vi "Master_continuous.vi"() -> ()   [LabVIEW 2021]
uses:
  Settings.ctl
  Control 2.ctl
  <vilib>/DAQmx/write.llb/DAQmx Write (Digital 1D U32 1Chan NSamp).vi
  <vilib>/DAQmx/create/channels.llb/DAQmx Create Channel (DO-Digital Output).vi
  <vilib>/DAQmx/configure/timing.llb/DAQmx Timing (Sample Clock).vi
  <vilib>/DAQmx/miscellaneous.llb/DAQmx Fill In Error Info.vi
panel:
  in  "stop":bool
  in  "Delay end (ms)":dbl=102.0
  out "# Samples":T1=7800.0 format="%#_9f"
  in  "Sampling Rate (Hz)":T1=100000.0 format="%#_9f"
  out "Blue LED":cluster{i32, dbl, dbl[]}(graph)={0, 1e-05, array[18000 elements]}
  out "EMCCD":cluster{i32, dbl, dbl[]}(graph)={0, 1e-05, array[18000 elements]}
  out "Whisker Cam":cluster{i32, dbl, dbl[]}(graph)={0, 1e-05, array[18000 elements]}
  out "Red LED":cluster{i32, dbl, dbl[]}(graph)={0, 1e-05, array[18000 elements]}
  out "Amber LED":cluster{i32, dbl, dbl[]}(graph)={0, 1e-05, array[18000 elements]}
  out "LSCI Sequence":cluster{i32, dbl, dbl[]}(graph)={0, 1e-05, array[18000 elements]}
  in  "Time Between (ms)":T2=1.5 format="%#_9f"
  in  "Red Exposure Width (ms)":T1=41.0 format="%#_9f"
  in  "Red Start (ms)":T1=120.0 format="%#_9f"
  in  "Frames/Seq":i32=12
  in  "Exposure Width (ms)":T1=5.0 format="%#_9f"
  in  "Blue Exposure Width [50-100] (ms)":T1=41.0 format="%#_9f"
  in  "Amber Start Time":T1=60.0 format="%#_9f"
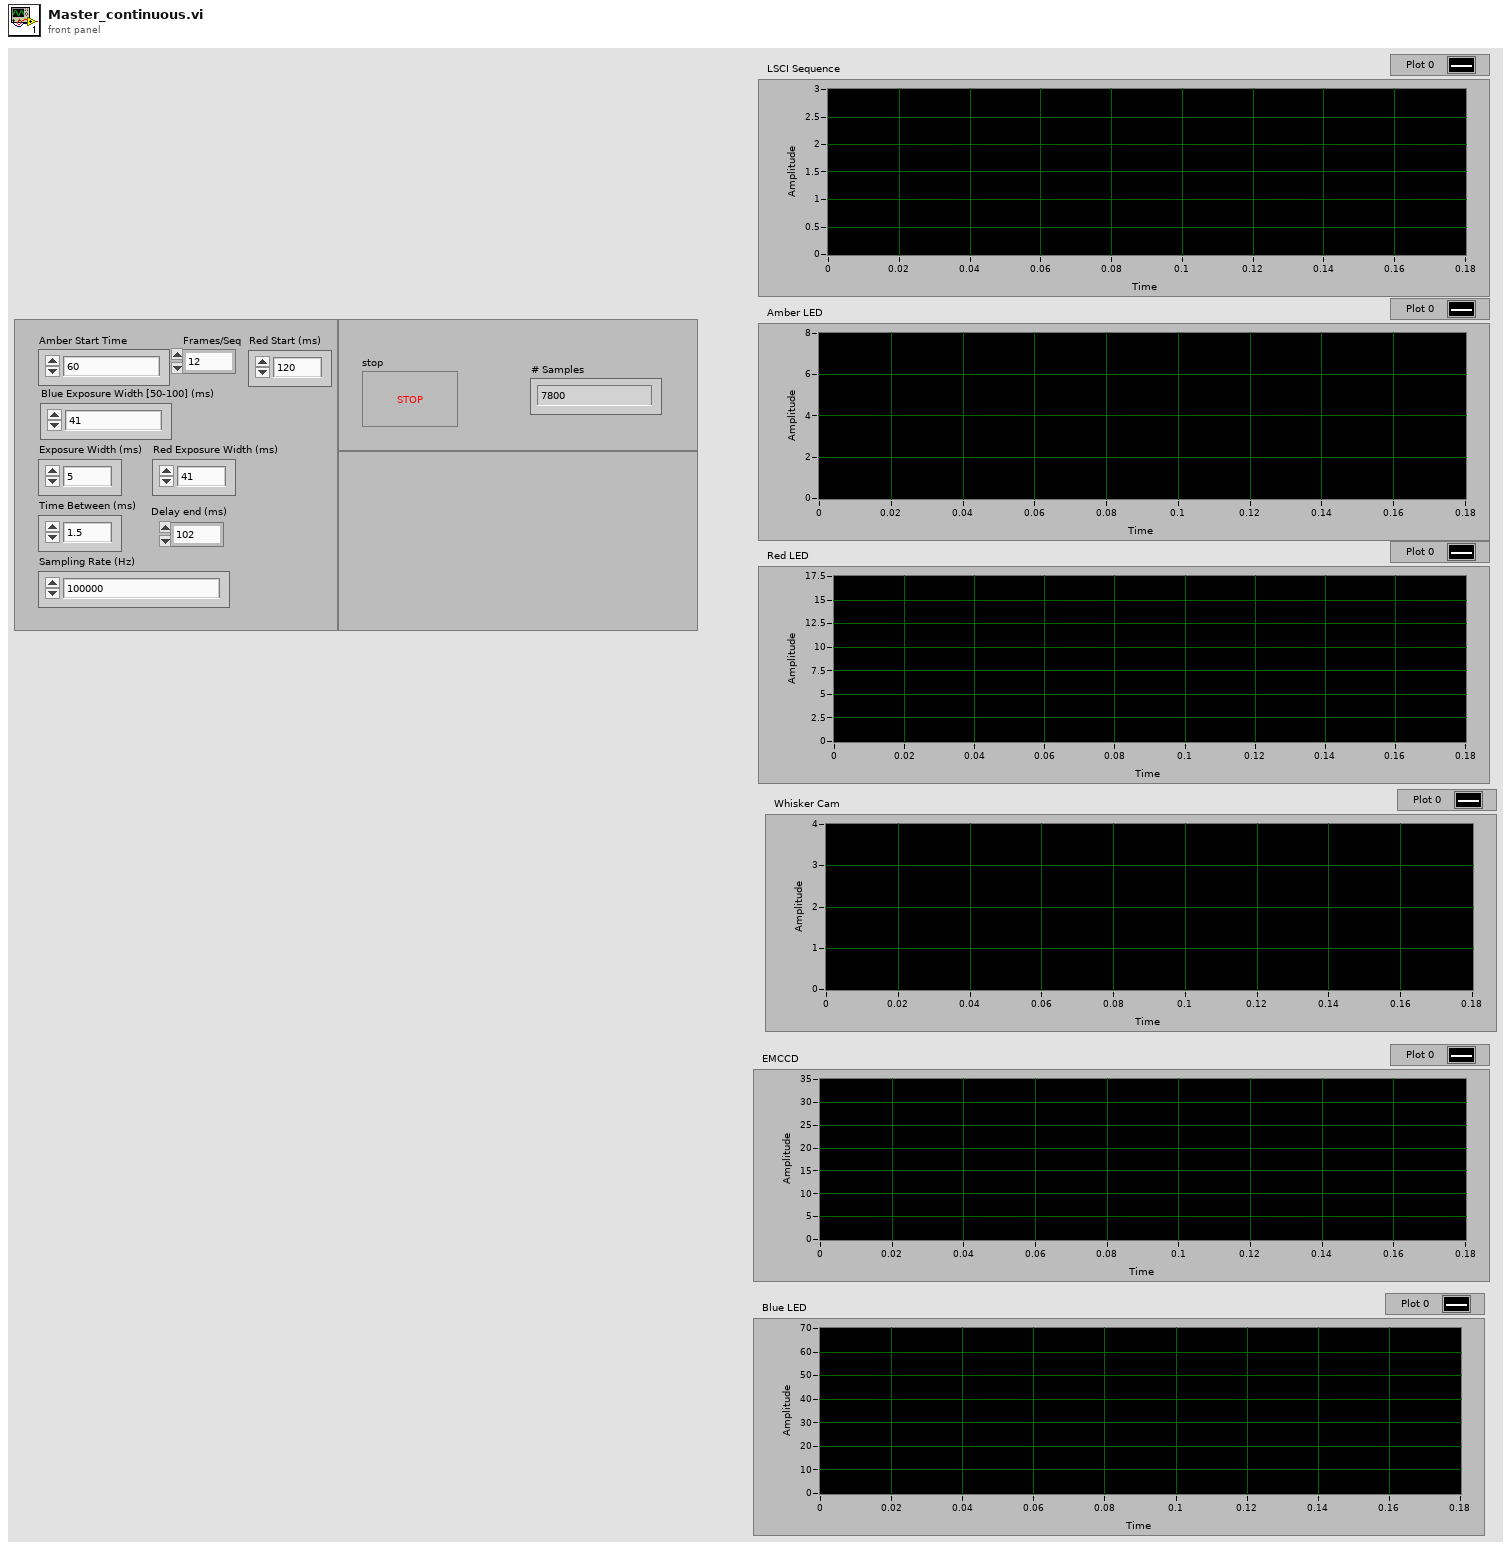
[diagram p1: front panel]
types:
  T1 = typedef "Settings.ctl" = dbl
  T2 = typedef "Control 2.ctl" = dbl
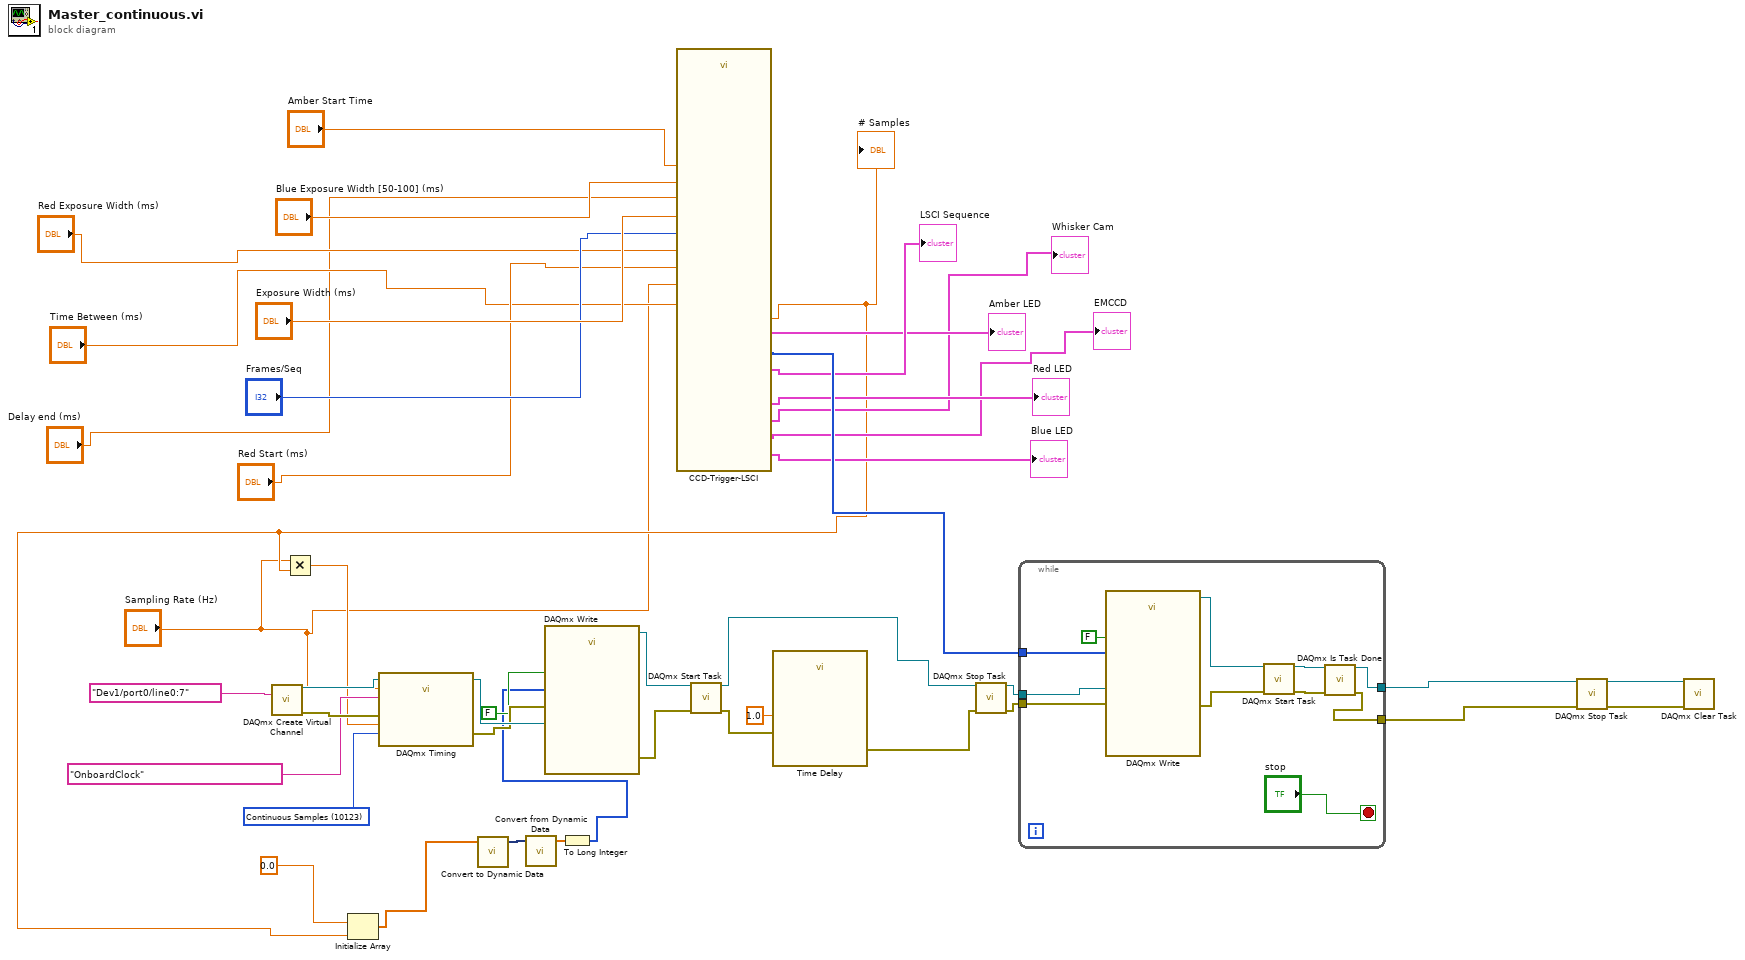
[diagram p0: block diagram]
diagram:
  w9 = 10123 items=["Finite Samples"=10178, "Continuous Samples"=10123, "Hardware Timed Single Point"=12522] ("sample mode")
  n1 = call-poly <vilib>:"DAQmx Create Virtual Channel.vi"("lines"=tag "Dev1/port0/line0:7") -> ("task out"=w26:refnum<k21>, "error out"=w25:errorcluster)  [unwired: 13 in]
  n2 = call "CCD-Trigger-LSCI.vi"("Frames/Seq"="Frames/Seq", "Exposure Width (ms) in"="Exposure Width (ms)", "Blue Exposure Width [50-100] (ms)"="Blue Exposure Width [50-100] (ms)", "Time Between (ms)"="Time Between (ms)", "Red Start Time"="Red Start (ms)", "Sampling Rate"="Sampling Rate (Hz)", "Amber Start Time"="Amber Start Time", "Red Exposure Width [50-80] (ms)"="Red Exposure Width (ms)", "Delay End (ms)"="Delay end (ms)") -> ("Blue LED"=→"Blue LED":cluster{i32, dbl, dbl[]}, "LSCI CCD"=→"LSCI Sequence":cluster{i32, dbl, dbl[]}, "Amber LED"=→"Amber LED":cluster{i32, dbl, dbl[]}, "Whisker Cam"=→"Whisker Cam":cluster{i32, dbl, dbl[]}, "EMCCD Trigger"=→"EMCCD":cluster{i32, dbl, dbl[]}, "Array out"=w33:u32[], "# Samples"=w14:T1, "Red LED"=→"Red LED":cluster{i32, dbl, dbl[]})  [unwired: 2 in, 1 out]
  "# Samples" <- w14
  n3 = Multiply(x="Sampling Rate (Hz)", y=w14) -> (x*y=w13:T1)
  n4 = Initialize Array(0.0 ("element"), w14) -> (w20:dbl[])
  n5 = call-poly <vilib>:"DAQmx Timing.vi"("task/channels in"=w26, "sample mode"=w9, "samples per channel"=w13, "rate"="Sampling Rate (Hz)", "source"=tag "OnboardClock", "error in"=w25) -> ("task out"=w19:refnum<k21>, "error out"=w18:errorcluster)  [unwired: 8 in]
  n6 = call "Convert to Dynamic Data"("Array"=w20) -> ("Dynamic Data Type"=w22:dynamicdata)  [unwired: 3 in]
  n7 = call "Convert from Dynamic Data"("Dynamic Data Type"=w22) -> ("Array"=w21:dbl[])  [unwired: 3 in]
  n8 = To Long Integer(number=w21) -> (32bit integer=w16:i32[])
  n9 = call-poly <vilib>:"DAQmx Write.vi"("task/channels in"=w19, "auto start"=FALSE, "data"=w16, "error in"=w18) -> ("task out"=w6:refnum<k21>, "error out"=w5:errorcluster)  [unwired: 9 in, 1 out]
  n10 = call <vilib>:"DAQmx Start Task.vi"("task/channels in"=w6, "error in"=w5) -> ("task out"=w2:refnum<k21>, "error out"=w4:errorcluster)  [unwired: 12 out]
  n11 = call "Time Delay"("error in (no error)"=w4, "Delay Time (s)"=1.0) -> ("error out"=w3:errorcluster)  [unwired: 9 in]
  n12 = call <vilib>:"DAQmx Stop Task.vi"("task/channels in"=w2, "error in"=w3) -> ("task out"=w11:refnum<k21>, "error out"=w12:errorcluster)  [unwired: 12 in]
  n13 = while {
    tunnel: [w47] -> w8
    tunnel: [w46] -> w7
    tunnel: w33 -> [w54]
    tunnel: w12 -> [w53]
    tunnel: w11 -> [w52]
    stop <- "stop" stop-if-true
    n14 = call-poly <vilib>:"DAQmx Write.vi"("task/channels in"=w52, "auto start"=FALSE, "data"=w54, "error in"=w53) -> ("task out"=w51:refnum<k21>, "error out"=w50:errorcluster)  [unwired: 9 in, 1 out]
    n15 = call <vilib>:"DAQmx Start Task.vi"("task/channels in"=w51, "error in"=w50) -> ("task out"=w49:refnum<k21>, "error out"=w48:errorcluster)  [unwired: 12 out]
    n16 = call <vilib>:"DAQmx Is Task Done.vi"("task/channels in"=w49, "error in"=w48) -> ("task out"=w47:refnum<k21>, "error out"=w46:errorcluster)  [unwired: 11 in, 1 out]
  }
  n17 = call <vilib>:"DAQmx Stop Task.vi"("task/channels in"=w8, "error in"=w7) -> ("task out"=w42:refnum<k21>, "error out"=w41:errorcluster)  [unwired: 12 in]
  n18 = call <vilib>:"DAQmx Clear Task.vi"("task in"=w42, "error in"=w41) -> ()  [unwired: 13 in, 1 out]
